vi "Epsilon.vi"(0 "Image":T2=refnum, 5 "SegImg":T2=refnum, 7 "Gyro Position":dbl=-19.9838407000004) -> ()   [LabVIEW 2016]
uses:
  <vilib>/vision/Image Controls.llb/IMAQ Image.ctl
  <vilib>/Rock Robotics/Network Tables/NT Read Boolean.vi
  AutoaimVar.vi
  <vilib>/Rock Robotics/Network Tables/NT Write Number.vi
  Robot Global Data.vi
  <vilib>/vision/NI_Vision_Development_Module.lvlib
panel:
  in  "Search Rect (entire image)":T1={"Left"=40, "Top"=70, "Right"=120, "Bottom"=230, "Rotation"=0.0} {"Rotation" format="%.2f"; "Left" scale=0.0..1024.0; "Right" scale=0.0..1024.0}
  out "segmented image 2":T2(plugin-control)
  in  "Residue Threshold 2":dbl=99999.0
  in  "Offset 2":dbl
  in  "B max 2":i32=255
  in  "B min 2":i32=149
  in  "G max 2":i32=255
  in  "G min 2":i32=20
  in  "R max 2":i32=128
  in  "R min 2":i32=123
  in  "Offset":dbl=3.5
  out "Error":dbl=3.248421790165897e-05
  out "XY Graph":cluster{dbl[], dbl[]}(graph)={[96.75, 96.46666717529297, 96.75, 96.75, 96.63636016845703, 96.75], [-19.966853120000398, -19.977255840000396, -19.979558560000395, -19.982435260000397, -19.973537980000398, -19.9838407000004]}
  out "Gyro Degrees":dbl[](array[numeric])=[-19.966853120000398, -19.977255840000396, -19.979558560000395, -19.982435260000397, -19.973537980000398, -19.9838407000004]
  out "Screen X":dbl[](array[numeric])=[96.75, 96.46666717529297, 96.75, 96.75, 96.63636016845703, 96.75]
  in  "Residue Threshold":dbl=99999.0
  out "segmented image":T2(plugin-control)
  in  "B max":i32=255
  in  "B min":i32=80
  in  "G max":i32=255
  in  "G min":i32=75
  in  "R max":i32=128
  in  "R min":i32=112
  out "Camera Image":T2(plugin-control)
  out "Objects":T3(array[cluster])=[{"Object Center"={"X"=96.75, "Y"=19.916666}, "Bounding Box"={"X Left"=96, "Y Top"=18, "X Right"=99, "Y Bottom"=23}, "Area"=12.0, "Orientation"=85.16332, "Aspect Ratio"=0.6, "Nb Holes"=0}] {"Aspect Ratio" format="%.2f"; "Orientation" format="%.2f"; "Area" format="%.2f"; "Object Center"."Y" format="%.2f"; "Object Center"."X" format="%.2f"}
  out "Image Out":T2
  out "Number of Objects":i32=1
  out "error out":errorcluster
  in  "error in (no error)":errorcluster
  in  "Settings":T4={"Objects"=0, "Threshold"=128, "Reject Border"=FALSE, "Fill Holes"=FALSE, "Min Object Size"=TRUE, "Min Size"=16, "Max Object Size"=FALSE, "Max Size"=100, "Show Search Area"=TRUE, "Show Center"=TRUE, "Show Bounding Box"=TRUE} {"Objects" items=["Bright Objects", "Dark Objects"]; "Threshold" min=1 max=999999999 step=1; "Max Size" min=1 max=999999999 step=1; "Min Size" min=1 max=999999999 step=1}
  # "Comp Bot Calibration"
  # "Proto Bot Calibration"
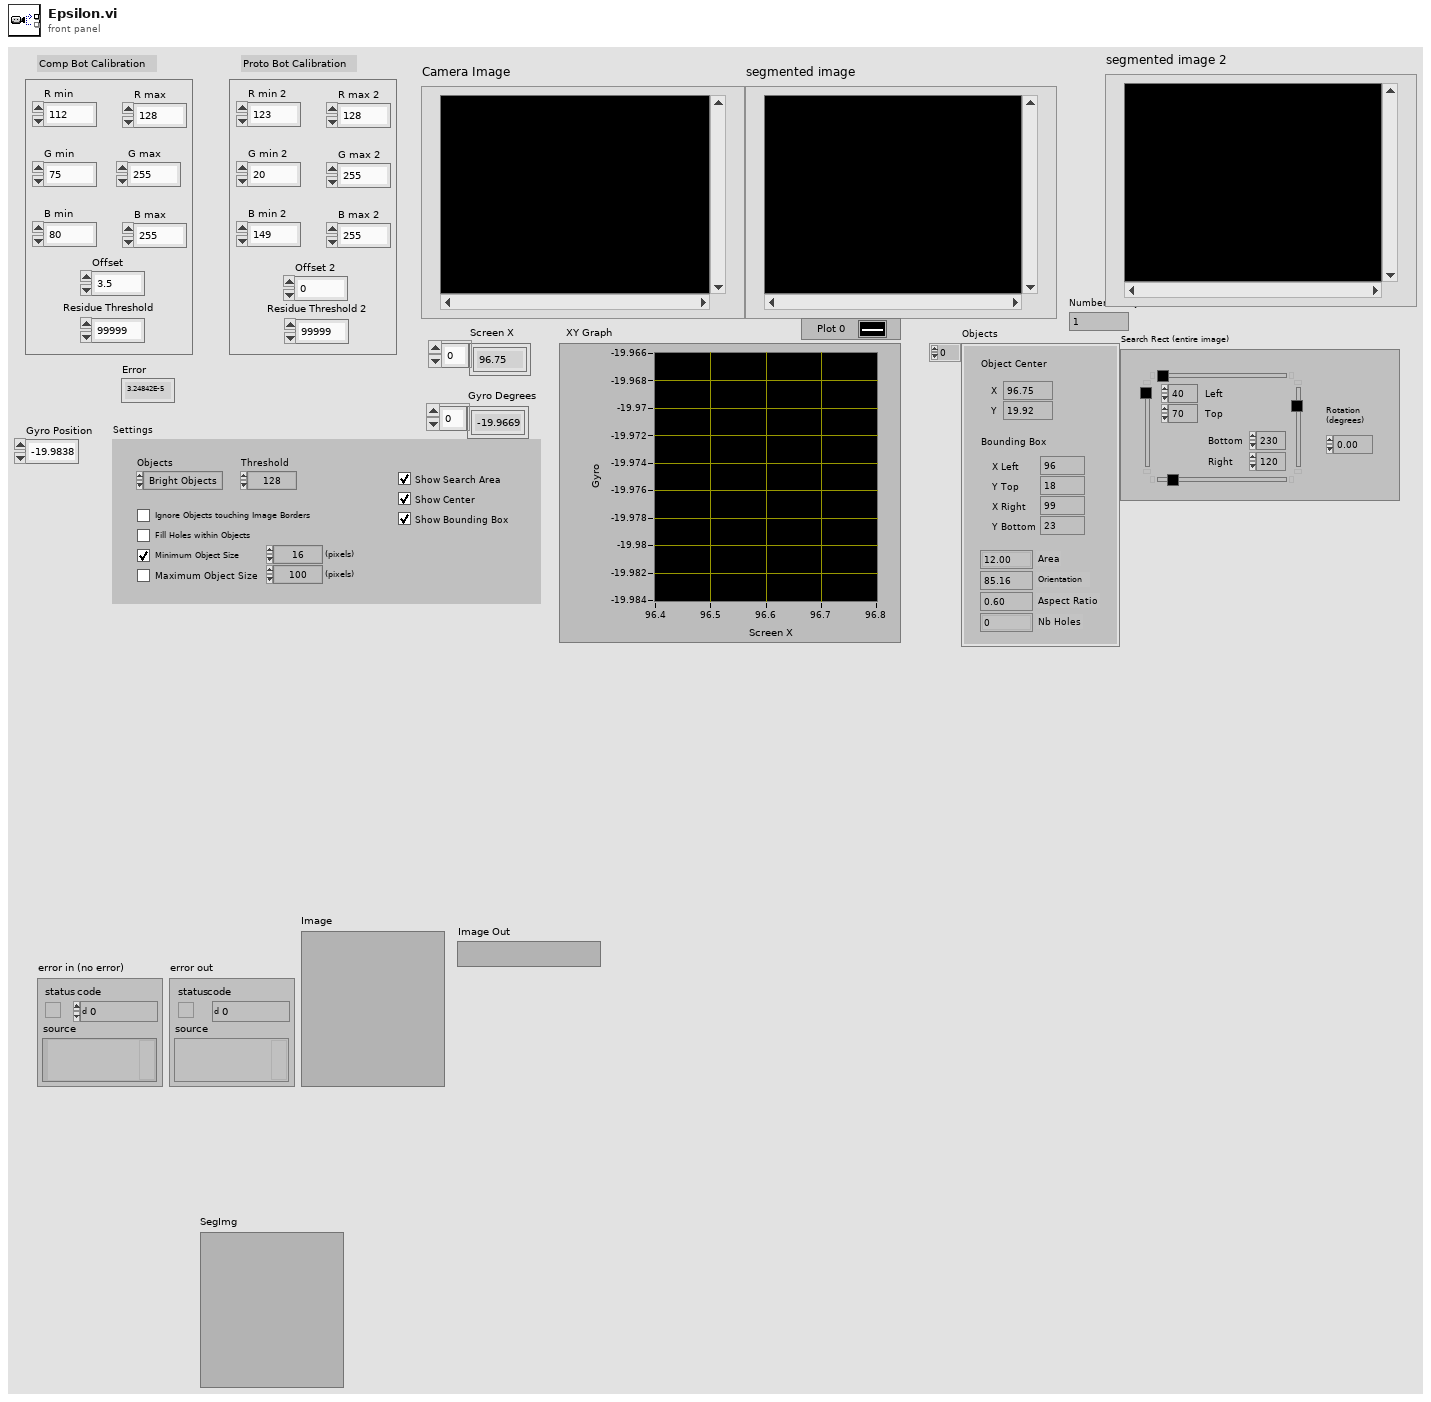
[diagram p1: front panel]
types:
  T1 = typedef "IMAQ Rectangle" = cluster{"Left":i32, "Top":i32, "Right":i32, "Bottom":i32, "Rotation":dbl}
  T2 = typedef "IMAQ Image.ctl" = refnum<image>
  T3 = cluster{"Object Center":cluster{"X":sgl, "Y":sgl}, "Bounding Box":cluster{"X Left":i32, "Y Top":i32, "X Right":i32, "Y Bottom":i32}, "Area":sgl, "Orientation":sgl, "Aspect Ratio":sgl, "Nb Holes":i32}[]
  T4 = cluster{"Objects":u16, "Threshold":i32, "Reject Border":bool, "Fill Holes":bool, "Min Object Size":bool, "Min Size":i32, "Max Object Size":bool, "Max Size":i32, "Show Search Area":bool, "Show Center":bool, "Show Bounding Box":bool}
  T5 = typedef "WPI_GyroDevRef.ctl" = cluster{"DevStatus":errorcluster, "Analog Channel":T6, "Offset":dbl, "Gain (VoltsPerDegree/Second)":dbl, "Gyro Type":enum16{"Analog", "XRS450"}, "Handle":i32, "SPI Bus":T7, "Device Found":bool, "Sample Rate":dbl, "Calibrate On Open":bool}
  T6 = typedef "FPGA_AIChannel.ctl" = enum8{"AI 0", "AI 1", "AI 2", "AI 3", "AI MXP 0", "AI MXP 1", "AI MXP 2", "AI MXP 3", "Invalid"}
  T7 = typedef "spi_bus.ctl" = enum16{"SPI On-Board, CS0", "SPI On-Board, CS1", "SPI On-Board, CS2", "SPI On-Board, CS3", "SPI MXP", "Invalid"}
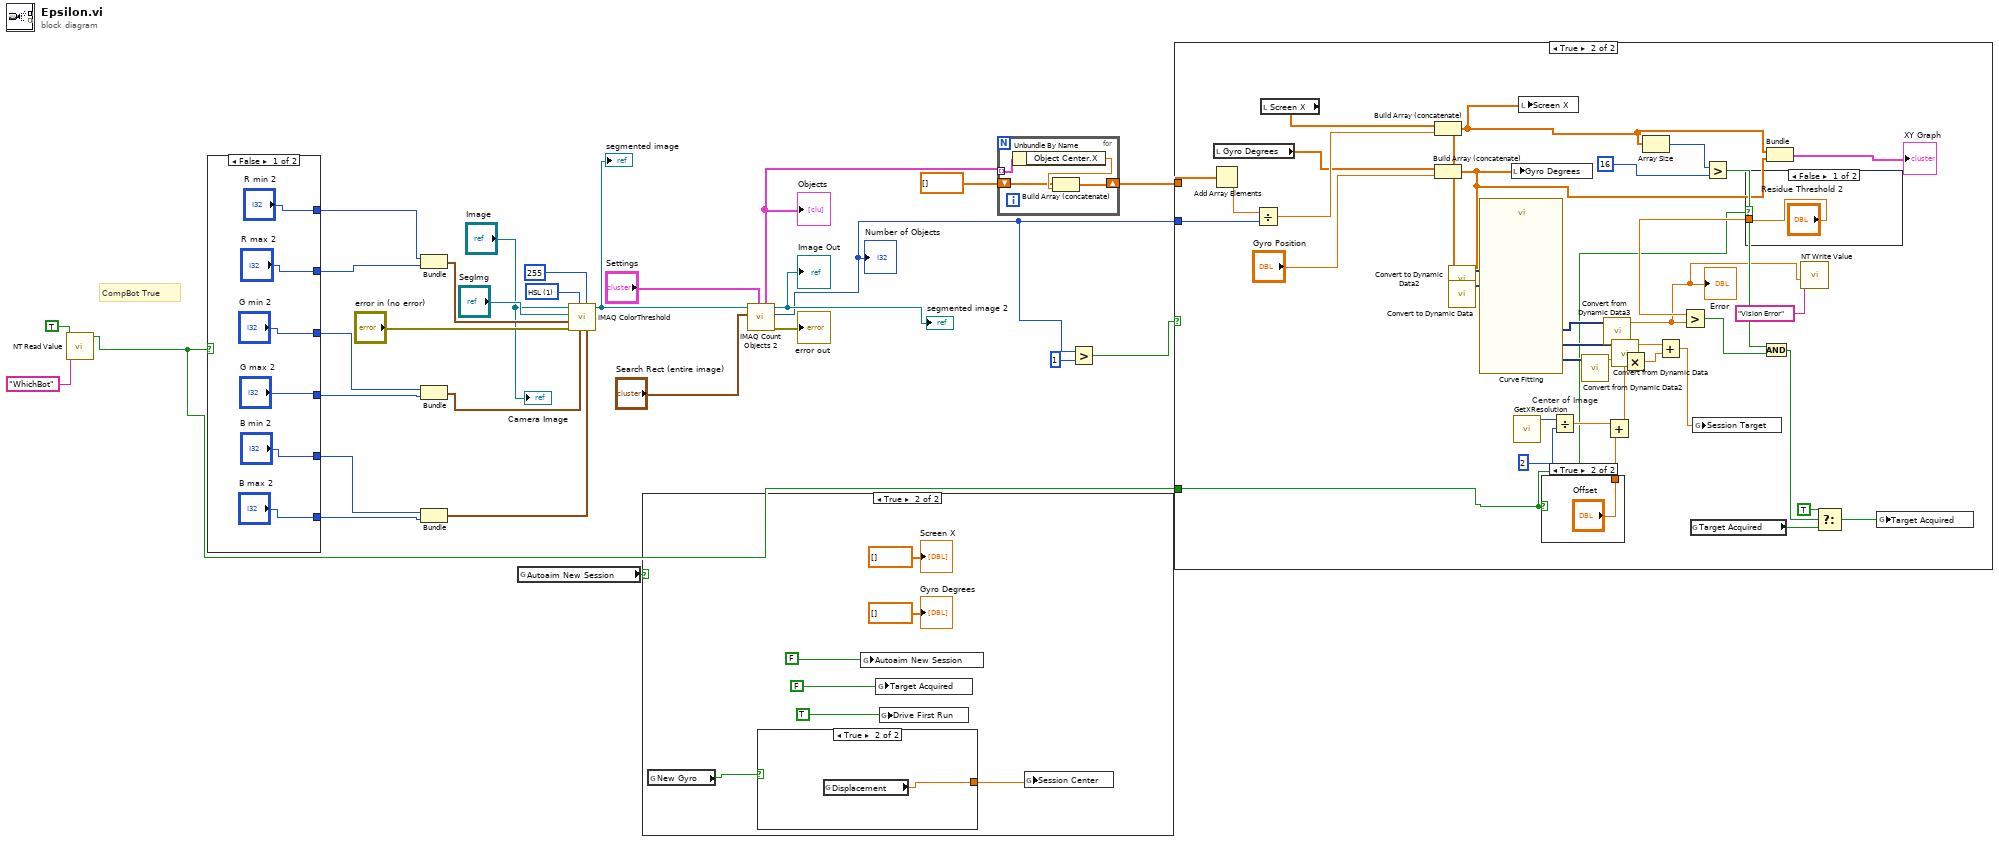
[diagram p0: block diagram]
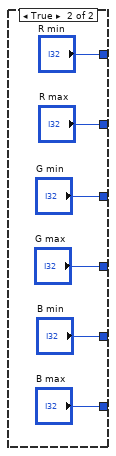
[diagram p2: hidden frame]
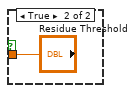
[diagram p4: hidden frame]
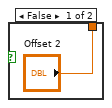
[diagram p5: hidden frame]
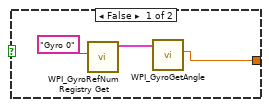
[diagram p7: hidden frame]
diagram:
  w15 = u16 1 items=["RGB", "HSL", "HSV", "HSI"] ("Color Mode")
  # "CompBot True"
  n1 = call-poly <vilib>:"NT Read Value.vi"("Default Value"=TRUE, "Name"="WhichBot") -> ("Boolean"=w7:bool)  [unwired: 8 in, 1 out]
  n2 = case shown="False" w7 {
    tunnel: ["G min 2" "G min"] -> w23
    tunnel: ["G max 2" "G max"] -> w22
    tunnel: ["B max 2" "B max"] -> w21
    tunnel: ["B min 2" "B min"] -> w20
    tunnel: ["R min 2" "R min"] -> w19
    tunnel: ["R max 2" "R max"] -> w18
    frame False {
    }
    frame True {
    }
  }
  n3 = Bundle("R min"=w19, "R max"=w18) -> (w29:cluster{"R min":i32, "R max":i32})  [unwired: 1 in]
  n4 = Bundle("G min"=w23, "G max"=w22) -> (w28:cluster{"G min":i32, "G max":i32})  [unwired: 1 in]
  n5 = Bundle("B min"=w20, "B max"=w21) -> (w24:cluster{"B min":i32, "B max":i32})  [unwired: 1 in]
  n6 = global read "AutoaimVar.vi" "Autoaim New Session"() -> (w10:bool)
  n7 = call "IMAQ ColorThreshold"("Blue or Luma or Val or Inten Range"=w24, "Replace Value"=255, "Green or Sat Range"=w28, "Color Mode"=w15, "error in (no error)"="error in (no error)", "Red or Hue Range"=w29, "Image Dst"="SegImg", "Image Src"="Image") -> ("Image Dst Out"=w14:T2)  [unwired: 2 in, 1 out]
  "segmented image" <- w14
  n8 = case shown="True" w10 {
    frame False {
    }
    frame True {
      n9 = global read "Robot Global Data.vi" "New Gyro"() -> (w43:bool)
      n10 = case shown="True" w43 {
        tunnel: [w49 w52] -> w42
        frame False {
          n11 = call <vilib>:"WPI_GyroRefNum Registry Get.vi"("refnum name"="Gyro 0") -> ("GyroDevRef"=w50:T5)  [unwired: 9 in, 1 out]
          n12 = call <vilib>:"WPI_GyroGetAngle.vi"("GyroDevRef"=w50) -> ("Angle"=w49:dbl)  [unwired: 6 in, 4 out]
        }
        frame True {
          n13 = global read "Robot Global Data.vi" "Displacement"() -> (w52:dbl)
        }
      }
      n14 = global write "AutoaimVar.vi" "Autoaim New Session"(FALSE) -> ()
      n15 = global write "AutoaimVar.vi" "Target Acquired"(FALSE ("Target Acquired")) -> ()
      n16 = global write "AutoaimVar.vi" "Drive First Run"(TRUE ("Drive First Run")) -> ()
      n17 = global write "AutoaimVar.vi" "Session Center"(w42) -> ()
      "Screen X" <- dbl[] [] ("Array")
      "Gyro Degrees" <- dbl[] [] ("Array 2")
    }
  }
  n18 = call "IMAQ Count Objects 2"("Settings"="Settings", "Search Rect (entire image)"="Search Rect (entire image)", "Image"=w14) -> ("error out"=→"error out":errorcluster, "Number of Objects"=w3:i32, "Image Out"=→"Image Out" →"segmented image 2":T2, "Objects"=w12:T3)  [unwired: 4 in, 1 out]
  "Number of Objects" <- w3
  "Objects" <- w12
  n19 = for {
    tunnel: w12 -> [w56] mode=indexing
    shift-right: [w54] -> w11
    shift-left: sgl[] [] -> [w53]
    n20 = Unbundle By Name(w56) -> ("Object Center.X"=w55:sgl)
    n21 = Build Array (concatenate)(w53, w55) -> (w54:sgl[])
  }
  n22 = Greater?(x=w3, y=1) -> (0:w1:bool)
  n23 = case shown="True" w1 {
    tunnel: w11 -> [_ w90]
    tunnel: w3 -> [_ w89]
    tunnel: w7 -> [_ w58]
    frame False {
    }
    frame True {
      n24 = local read "Gyro Degrees"() -> (w85:dbl[])
      n25 = Add Array Elements(numeric array=w90) -> (sum=w88:sgl)
      n26 = Divide(x=w88, y=w89) -> (x/y=w86:sgl)
      n27 = local read "Screen X"() -> (w87:dbl[])
      n28 = Build Array (concatenate)(w87, w86) -> (w69:dbl[])
      n29 = Build Array (concatenate)(w85, "Gyro Position") -> (w68:dbl[])
      n30 = call "Convert to Dynamic Data2"("Array"=w68) -> ("Dynamic Data Type"=w83:dynamicdata)  [unwired: 3 in]
      n31 = call "Convert to Dynamic Data"("Array"=w69) -> ("Dynamic Data Type"=w84:dynamicdata)  [unwired: 3 in]
      n32 = call "Curve Fitting"("Locations"=w84, "Signals"=w83) -> ("mean squared error"=w66:dynamicdata, "slope"=w82:dynamicdata, "intercept"=w80:dynamicdata)  [unwired: 4 in, 3 out]
      n33 = local write "Gyro Degrees"(w68) -> ()
      n34 = call "GetXResolution.vi"() -> ("x+y"=w91:i32)  [unwired: 11 in]
      n35 = local write "Screen X"(w69) -> ()
      n36 = case shown="True" w58 {
        tunnel: ["Offset 2" "Offset"] -> w60
        frame False {
        }
        frame True {
        }
      }
      n37 = Divide "Center of Image"(x=w91, y=2) -> (x/y=w61:dbl)
      n38 = call "Convert from Dynamic Data2"("Dynamic Data Type"=w82) -> ("Scalar"=w81:dbl)  [unwired: 3 in]
      n39 = call "Convert from Dynamic Data3"("Dynamic Data Type"=w66) -> ("Scalar"=w63:dbl)  [unwired: 3 in]
      "Error" <- w63
      n40 = Add(x=w61, y=w60) -> (x+y=w59:dbl)
      n41 = call "Convert from Dynamic Data"("Dynamic Data Type"=w80) -> ("Scalar"=w79:dbl)  [unwired: 3 in]
      n42 = Multiply(x=w81, y=w59) -> (x*y=w78:dbl)
      n43 = Array Size(array=w69) -> (size(s)=w77:i32)
      n44 = Add(x=w79, y=w78) -> (x+y=w70:dbl)
      n45 = global read "AutoaimVar.vi" "Target Acquired"() -> (w72:bool)
      n46 = global write "AutoaimVar.vi" "Session Target"(w70) -> ()
      n47 = Greater?(x=w77, y=16) -> (0:w76:bool)
      n48 = case shown="False" w58 {
        tunnel: ["Residue Threshold 2" "Residue Threshold"] -> w65
        frame False {
        }
        frame True {
        }
      }
      n49 = Greater?(x=w65, y=w63) -> (0:w75:bool)
      n50 = And(x=w76, y=w75) -> (x .and. y?=w74:bool)
      n51 = Bundle(w69, w68) -> (→"XY Graph":cluster{dbl[], dbl[]})  [unwired: 1 in]
      n52 = call-poly <vilib>:"NT Write Value.vi"("Numeric"=w63, "Name"="Vision Error") -> ()  [unwired: 9 in, 1 out]
      n53 = Select(t=TRUE, s=w74, f=w72) -> (s? t:f=w71:bool)
      n54 = global write "AutoaimVar.vi" "Target Acquired"(w71) -> ()
    }
  }
  "Camera Image" <- "Image"
